vi "PH_Close.vi"(0 "devidx":i32) -> ()   [LabVIEW 2019]
uses:
  phlib64.dll
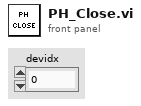
[diagram p1: front panel]
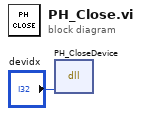
[diagram p0: block diagram]
diagram:
  n1 = dll-call lib="C:/Users/manip/Documents/Controle_Manip_2020/subVIs/PicoHarp/phlib64.dll" fn="PH_CloseDevice"("devidx"="devidx") -> ()  [unwired: 5 in, 2 out]
